vi "Off.vi"(8 "error in (no error)":errorcluster, 11 "SimPump in":refnum<class "SimPump.lvclass">) -> (0 "error out":errorcluster, 3 "SimPump out":refnum<class "SimPump.lvclass">)   [LabVIEW 2019, in "SimPump.lvclass"]
doc: "Turns the pump off.\n\nwww.sciware.com.au"
uses:
  SimPump.lvclass
  Private/CmdQueueType.ctl
  SimPump.lvclass/SimPump.ctl
panel:
  # "BSD License (http://www.opensource.org/licenses/bsd-license.php)"
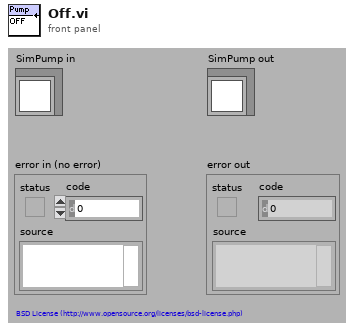
[diagram p1: front panel]
types:
  T1 = typedef "SimPump.lvclass/CmdQueueType.ctl" = string
  T2 = typedef "SimPump.lvclass/CmdQueueRef.ctl" = refnum<queue>
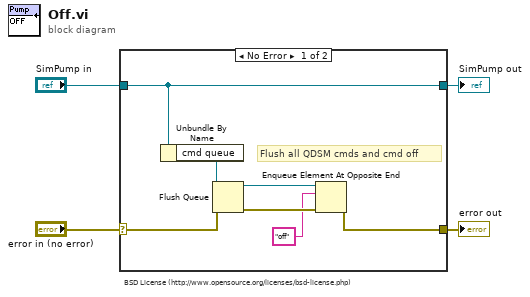
[diagram p0: block diagram]
diagram:
  # "BSD License (http://www.opensource.org/licenses/bsd-license.php)"
  n1 = case shown="No Error" "error in (no error)" {
    selector: "error in (no error)" -> [w7 w13]
    tunnel: [w6 w13] -> w3
    tunnel: [w8 w12] -> w1
    tunnel: "SimPump in" -> [w8 w12]
    frame No Error {
      # "Flush all QDSM cmds and cmd off"
      n2 = Unbundle By Name(w8) -> ("cmd queue"=w11:T2)
      n3 = Flush Queue(queue=w11, error in (no error)=w7) -> (queue out=w9:T2, error out=w10:errorcluster)  [unwired: 1 out]
      n4 = Enqueue Element At Opposite End(queue=w9, element=T1 "off", error in (no error)=w10) -> (error out=w6:errorcluster)  [unwired: 1 in, 2 out]
    }
    frame Error {
    }
  }
  "error out" <- w3
  "SimPump out" <- w1
